vi "Point&Path@TransPlaceSnap__Parameter.vi"(1 "ParamterIn":string) -> (0 "ParamterOut":string)   [LabVIEW 2020]
panel:
  in  "IMAQ":string(combo)
  in  "MotorName":string(combo)
  in  "CrdCM":string(combo)
  in  "CrdPLSN":string(combo)
  in  "Confirm":bool
  # "Point&Path@TransPlaceSnap $Motor,$CrdPLSN,$CrdCamMotor,$ImaqPoint\n$Motor=Present Motion Position OR Relative Motion Position\n$ImaqPoint = Result\n$CrdPLSN: \n                  $CrdPLSN[0]=Motion Place Positon\n                  $CrdPLSN[1]= Snap Motion Positon\n                  $CrdPLSN[2] = PatternMatch IMAQ Position\n$CrdCamMotor:\n                  $CrdCamMotor[0] =Motion Positon at IMAQ Original\n                  $CrdCamMotor[1] =Motion Positon at IMAQ X Axis\n                  $CrdCamMotor[2] =Motion Positon at IMAQ Y Axis\n$ImaqPoint: IMAQ PaternMatch Position"
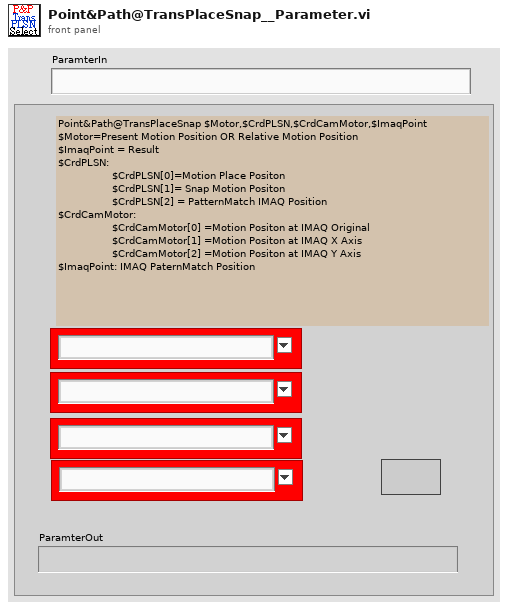
[diagram p1: front panel]
types:
  T1 = enum16{"Get", "UpdatePointS", "Init", "UpdateIndex", "GetCurrent&Index+1", "GetWithIndex", "ChkLast", "GetCurrent"}
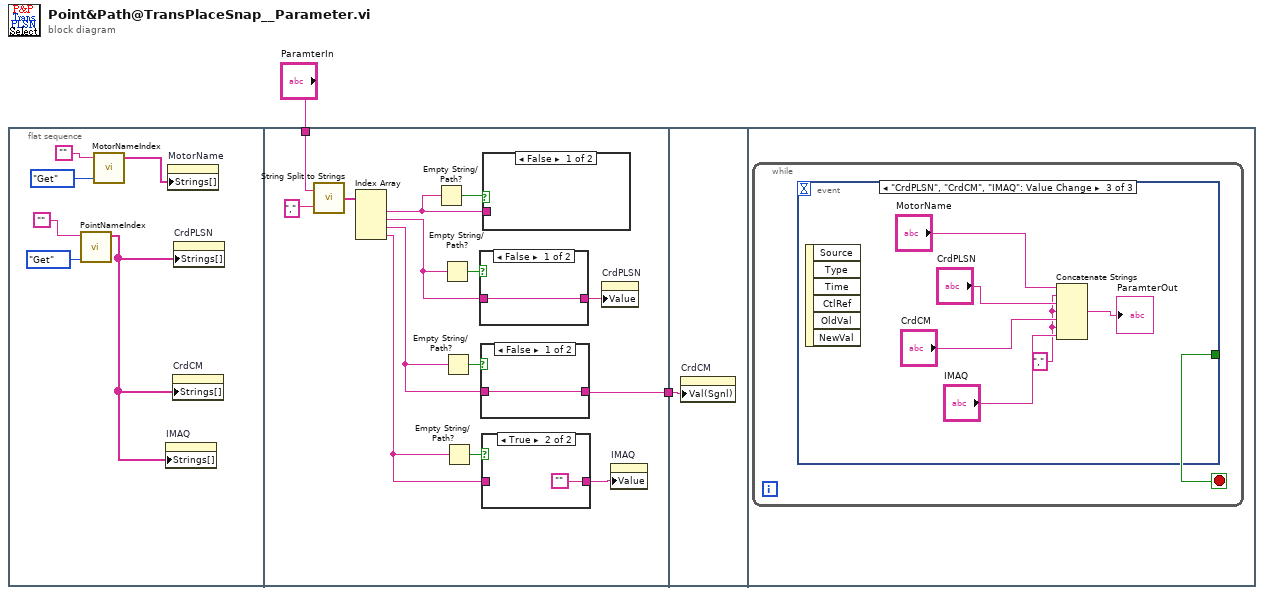
[diagram p0: block diagram]
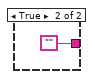
[diagram p3: hidden frame]
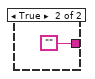
[diagram p4: hidden frame]
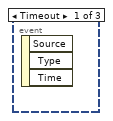
[diagram p6: hidden frame]
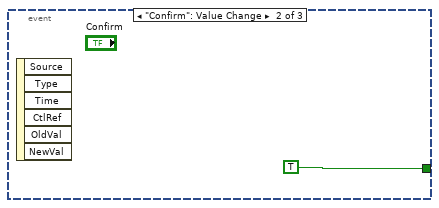
[diagram p7: hidden frame]
diagram:
  n1 = flat-sequence {
    tunnel: "ParamterIn" -> [w18]
    tunnel: [w12] -> w1
    tunnel: w1 -> [w29]
    frame #0 {
      n2 = call "PointNameIndex.vi"("OP"=T1."Get", "PointName"="") -> ("PointNameList"=w3:string[])  [unwired: 4 in, 5 out]
      n3 = call "MotorNameIndex.vi"("OP"=enum16{"Get", "Update", "Init"}."Get", "MotorName"="") -> ("MotorList"=w4:string[])  [unwired: 1 in, 2 out]
      n4 = property on="IMAQ" class="CmbBox"("Strings[]"=w3) -> ()  [unwired: 2 in, 2 out]
      n5 = property on="MotorName" class="CmbBox"("Strings[]"=w4) -> ()  [unwired: 2 in, 2 out]
      n6 = property on="CrdCM" class="CmbBox"("Strings[]"=w3) -> ()  [unwired: 2 in, 2 out]
      n7 = property on="CrdPLSN" class="CmbBox"("Strings[]"=w3) -> ()  [unwired: 2 in, 2 out]
    }
    frame #1 {
      n8 = call "String Split to Strings.vi"("search string/char (-)"=",", "String"=w18) -> ("Array"=w19:string[])
      n9 = Index Array(array=w19) -> (element #1=w17:string, element #2=w16:string, element #3=w13:string, element #4=w10:string)  [unwired: 4 in]
      n10 = Empty String/Path?(string/path=w17) -> (empty?=w22:bool)
      n11 = Empty String/Path?(string/path=w16) -> (empty?=w21:bool)
      n12 = Empty String/Path?(string/path=w13) -> (empty?=w14:bool)
      n13 = Empty String/Path?(string/path=w10) -> (empty?=w11:bool)
      n14 = case shown="False" w21 {
        tunnel: [w27 ""] -> w15
        tunnel: w16 -> [w27 _]
        frame False {
        }
        frame True {
        }
      }
      n15 = case shown="False" w14 {
        tunnel: [w25 ""] -> w12
        tunnel: w13 -> [w25 _]
        frame False {
        }
        frame True {
        }
      }
      n16 = case shown="True" w11 {
        tunnel: [w23 ""] -> w9
        tunnel: w10 -> [w23 _]
        frame False {
        }
        frame True {
        }
      }
      n17 = case shown="False" w22 {
        tunnel: w17 -> [_ _]
        frame False {
        }
        frame True {
        }
      }
      n18 = property on="CrdPLSN" class="CmbBox"("Value"=w15) -> ()  [unwired: 2 in, 2 out]
      n19 = property on="IMAQ" class="CmbBox"("Value"=w9) -> ()  [unwired: 2 in, 2 out]
    }
    frame #2 {
      n20 = property on="CrdCM" class="CmbBox"("Val(Sgnl)"=w29) -> ()  [unwired: 2 in, 2 out]
    }
    frame #3 {
      n21 = while {
        stop <- w30 stop-if-true
        n22 = event shown="[2] \"CrdPLSN\", \"CrdCM\", \"IMAQ\": Value Change" {
          selector: _ -> [_ _ _]
          dyn-events: _ -> [_ _ _]
          timeout: _ -> [_ _ _]
          tunnel: [_ TRUE _] -> w30
          event Timeout {
            n23 = event-data() -> ()  [unwired: 1 in, 3 out]
          }
          event "Confirm": Value Change {
            n24 = event-data() -> ()  [unwired: 1 in, 6 out]
          }
          event "CrdPLSN", "CrdCM", "IMAQ": Value Change {
            w32 = ","
            n25 = event-data() -> ()  [unwired: 1 in, 6 out]
            n26 = Concatenate Strings("MotorName", w32, "CrdPLSN", w32, "CrdCM", w32, "IMAQ") -> (→"ParamterOut":string)
          }
        }
      }
    }
  }
